vi "New Fixture.vi"() -> ()   [LabVIEW 2011]
panel:
  out "u2":bool
  out "update_1":string
  out "path_ref":refnum<vi>[](array[refnum])
  out "fixture_read":string
  out "fileexist":bool
  out "fixture":string
  out "3":bool
  out "2":bool
  out "1":bool
  in  "S4P40G":string
  in  "S4P27G":string
  in  "S4P20G":string
  out "graph_ref":refnum<vi>[](array[refnum])
  out "str_ref":refnum<vi>[](array[refnum])
  in  "S4P10G":string
  in  "Tap":enum32{"General", "Fixture Information"}(tab)
  in  "S4P Save?":bool
  in  "Rev:":string="A"
  in  "PCBPN:":string="120-000006H-048R"
  in  "Owner:":string="Shuangfeng yuan"
  in  "LifeCycle: (次)":string="3000"
  in  "Query":bool
  in  "Update":bool
  in  "Delete":bool
  in  "Save":bool
  in  "Local":bool
  in  "FixtureNo:":string="SFP+ 002"
  in  "Type:":string="SFP+"
  in  "Fixture Description:":string="SFP+ Cable Evaluation Board"
  in  "Count:":string="0"
  in  "Summary:":string
  in  "Excute":bool
  in  "40G":path
  in  "27G":path
  in  "20G":path
  in  "10G":path
  out "Delay(ns)":dbl
  in  "From File":bool
  out "Delay":T1(graph)
  out "Insertion Loss":T1(graph)
  in  "Count(invisible)":string
  in  "FixtureType":string
  in  "FixtureNo":string
  in  "FixtureRev":string
  in  "Import_FixS4P":bool caption="Start Test"
  in  "Port Type":u16(ring)
  # "SI Testing Fixture Management"
  # "Rev 1.1"
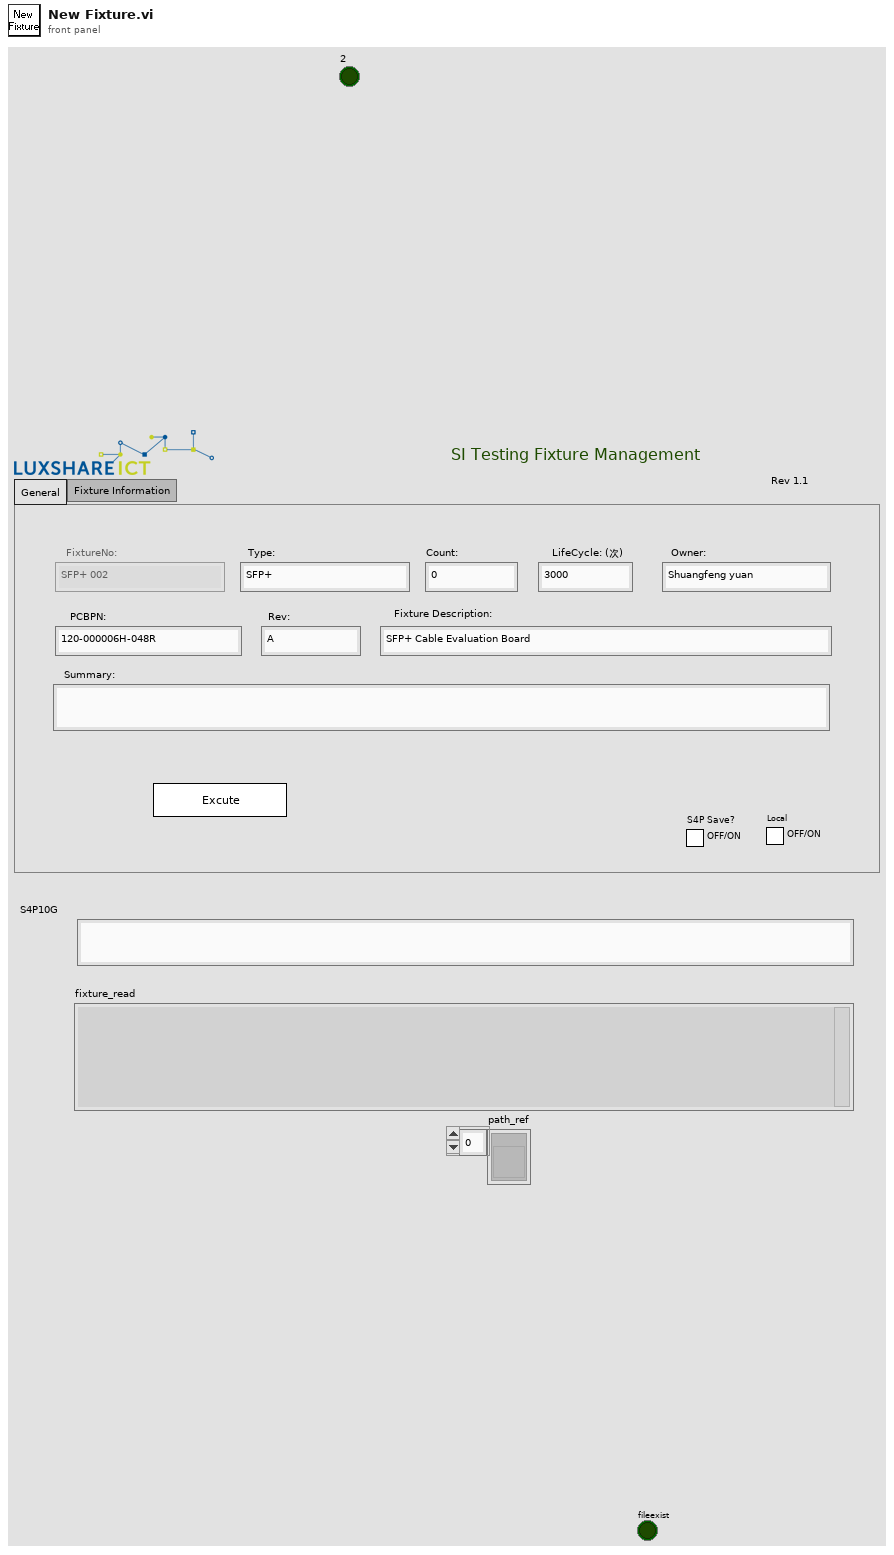
[diagram p1: front panel]
types:
  T1 = cluster{"Frequency(Hz)":dbl[], "Diff S-parameters Data":dbl[]}
  T2 = enum8{"Enabled", "Disabled", "Disabled and Grayed Out"}
  T3 = enum16{"查询表名", "查询列名", "查询记录", "查询总记录", "查询数据", "转换数据"}
  T4 = enum16{"big-endian, network order", "native, host order", "little-endian"}
  T5 = enum16{"", "创建表", "删除表", "添加表列", "删除表列", "添加数据", "删除数据"}
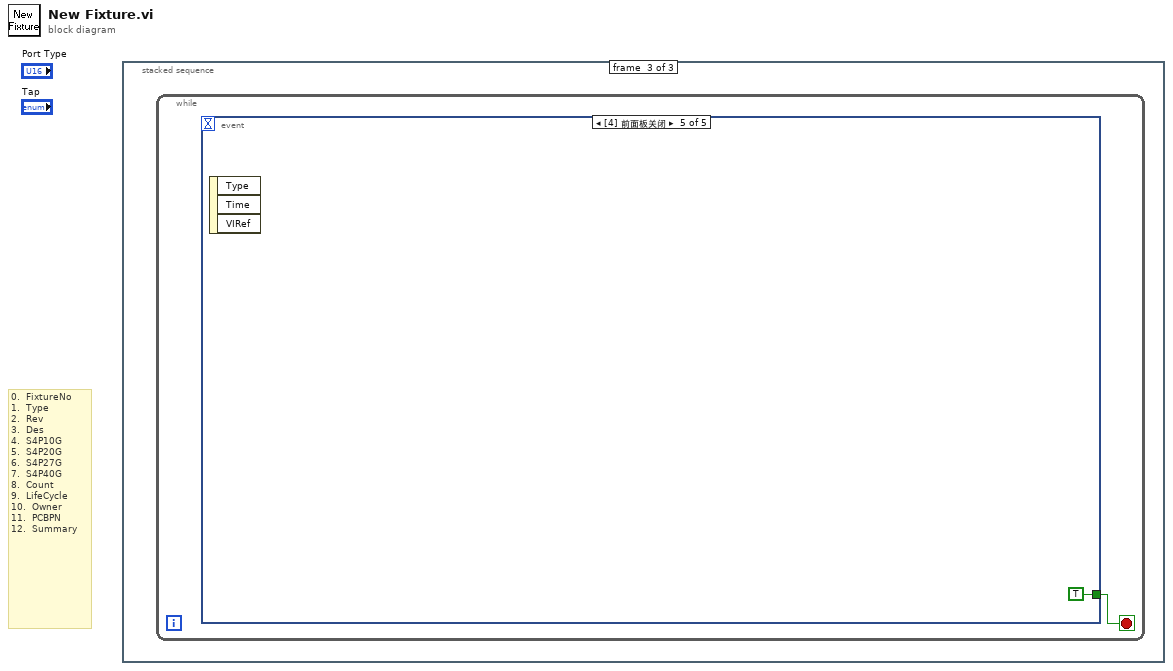
[diagram p0: block diagram]
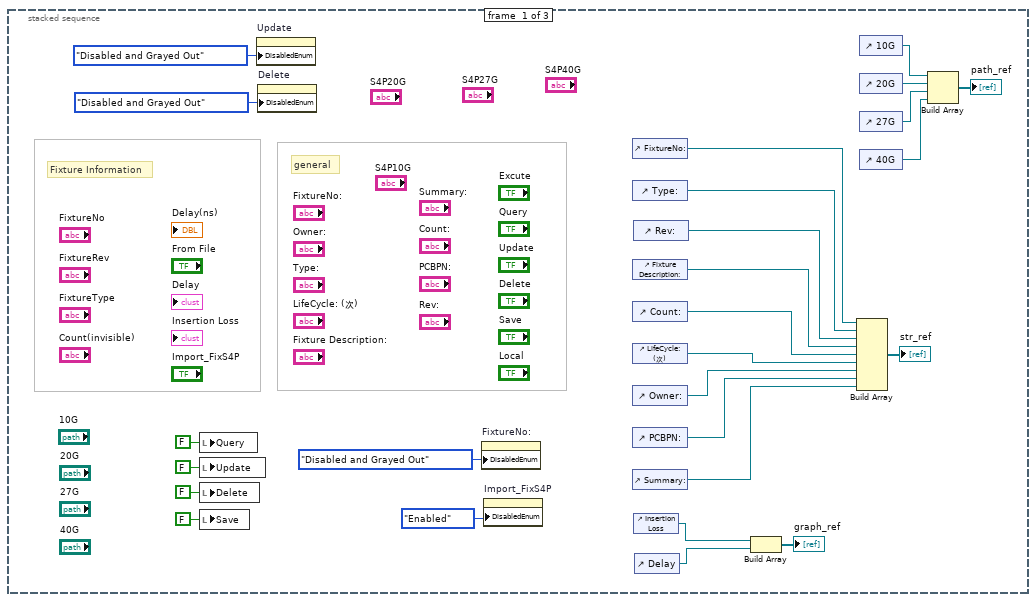
[diagram p2: hidden frame]
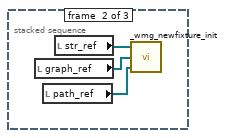
[diagram p3: hidden frame]
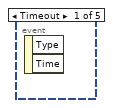
[diagram p4: hidden frame]
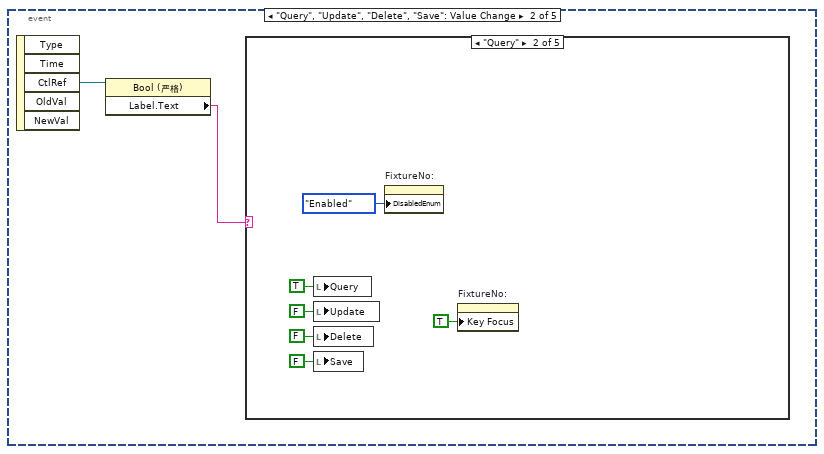
[diagram p5: hidden frame]
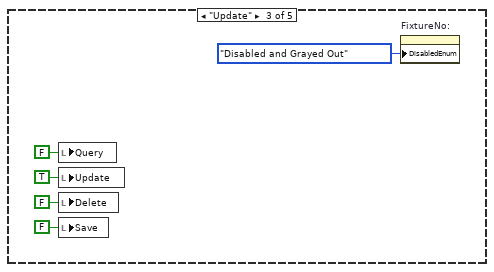
[diagram p7: hidden frame]
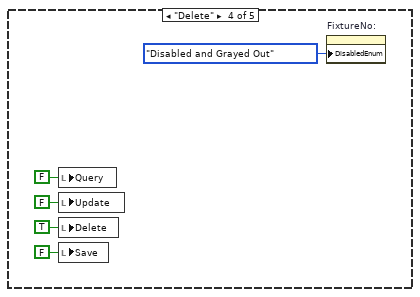
[diagram p8: hidden frame]
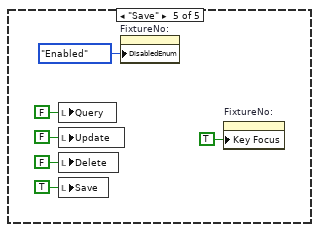
[diagram p9: hidden frame]
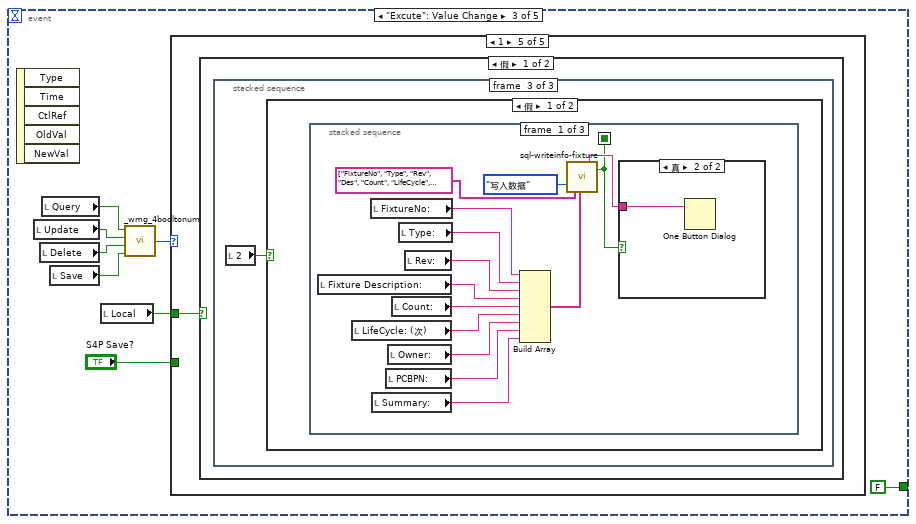
[diagram p10: hidden frame]
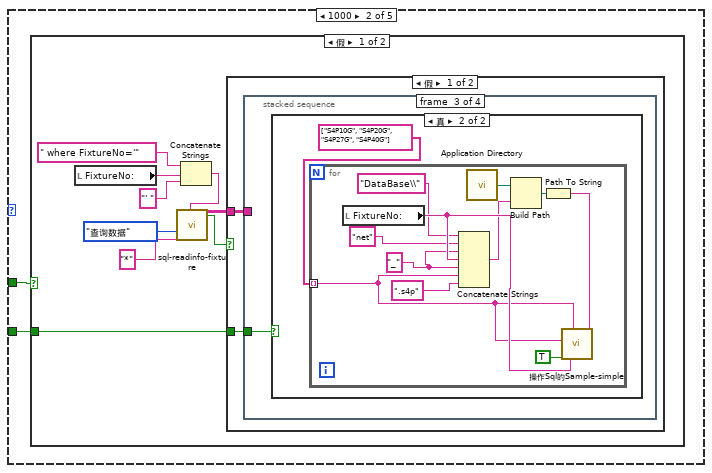
[diagram p12: hidden frame]
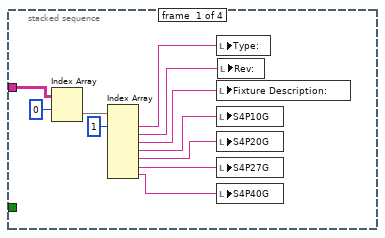
[diagram p13: hidden frame]
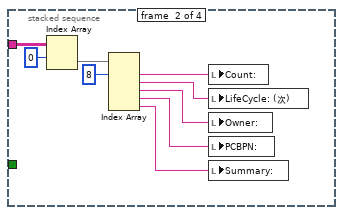
[diagram p14: hidden frame]
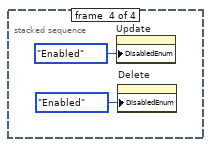
[diagram p16: hidden frame]
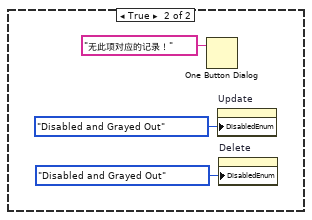
[diagram p17: hidden frame]
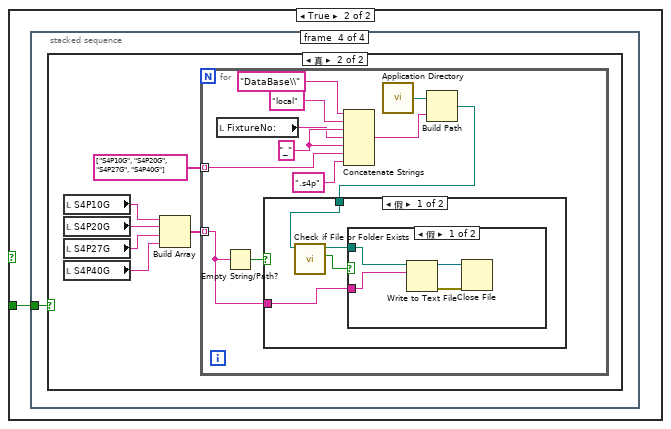
[diagram p18: hidden frame]
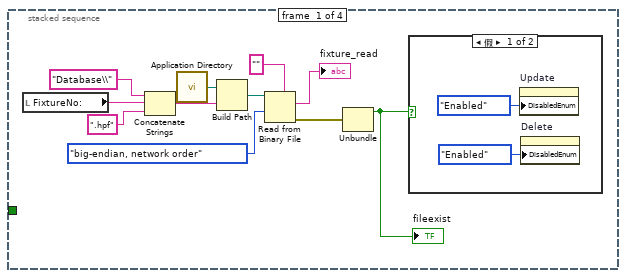
[diagram p19: hidden frame]
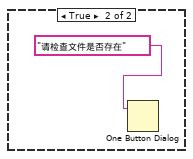
[diagram p20: hidden frame]
diagram:
  # "0.  FixtureNo\n1.  Type\n2.  Rev\n3.  Des\n4.  S4P10G\n5.  S4P20G\n6.  S4P27G\n7.  S4P40G\n8.  Count\n9.  LifeCycle\n10.  Owner\n11.  PCBPN\n12.  Summary"
  n1 = stacked-sequence {
    frame #0 {
      # "Fixture Information"
      # "general"
      n2 = local write "Query"(FALSE ("Query")) -> ()
      n3 = local write "Update"(FALSE ("Update")) -> ()
      n4 = local write "Delete"(FALSE ("Delete")) -> ()
      n5 = local write "Save"(FALSE ("Save")) -> ()
      n6 = property on="Update" class="Bool (严格)"("DisabledEnum"=T2."Disabled and Grayed Out" ("禁用")) -> ()  [unwired: 2 in, 2 out]
      n7 = property on="Delete" class="Bool (严格)"("DisabledEnum"=T2."Disabled and Grayed Out" ("禁用")) -> ()  [unwired: 2 in, 2 out]
      n8 = property on="FixtureNo:" class="Str"("DisabledEnum"=T2."Disabled and Grayed Out" ("禁用")) -> ()  [unwired: 2 in, 2 out]
      n9 = property on="Import_FixS4P" class="Bool"("DisabledEnum"=T2."Enabled" ("禁用")) -> ()  [unwired: 2 in, 2 out]
      n10 = control-ref of="FixtureNo:"() -> (w5:refnum<vi>)
      n11 = control-ref of="Type:"() -> (w4:refnum<vi>)
      n12 = control-ref of="Fixture Description:"() -> (w26:refnum<vi>)
      n13 = control-ref of="Count:"() -> (w25:refnum<vi>)
      n14 = control-ref of="LifeCycle: (次)"() -> (w24:refnum<vi>)
      n15 = control-ref of="Owner:"() -> (w23:refnum<vi>)
      n16 = control-ref of="PCBPN:"() -> (w22:refnum<vi>)
      n17 = control-ref of="Summary:"() -> (w21:refnum<vi>)
      n18 = control-ref of="Rev:"() -> (w3:refnum<vi>)
      n19 = control-ref of="Insertion Loss"() -> (w18:refnum<vi>)
      n20 = control-ref of="Delay"() -> (w17:refnum<vi>)
      n21 = Build Array(w18, w17) -> (→"graph_ref":refnum<vi>[])
      n22 = Build Array(w5, w4, w3, w26, w25, w24, w23, w22, w21) -> (→"str_ref":refnum<vi>[])
      n23 = control-ref of="10G"() -> (w10:refnum<vi>)
      n24 = control-ref of="20G"() -> (w9:refnum<vi>)
      n25 = control-ref of="27G"() -> (w8:refnum<vi>)
      n26 = control-ref of="40G"() -> (w7:refnum<vi>)
      n27 = Build Array(w10, w9, w8, w7) -> (→"path_ref":refnum<vi>[])
    }
    frame #1 {
      n28 = local read "graph_ref"() -> (w29:refnum<vi>[])
      n29 = local read "path_ref"() -> (w27:refnum<vi>[])
      n30 = local read "str_ref"() -> (w28:refnum<vi>[])
      n31 = call "_wmg_newfixture_init.vi"("path_ref"=w27, "graph_ref"=w29, "str_ref"=w28) -> ()  [unwired: 1 in]
    }
    frame #2 {
      n32 = while {
        stop <- w30 stop-if-true
        n33 = event shown="[4] 前面板关闭" {
          selector: _ -> [_ _ _ _ _]
          dyn-events: _ -> [_ _ _ _ _]
          timeout: _ -> [_ _ _ _ _]
          tunnel: [_ _ FALSE _ TRUE] -> w30
          event Timeout {
            n34 = event-data() -> ()  [unwired: 1 in, 2 out]
          }
          event "Query", "Update", "Delete", "Save": Value Change {
            n35 = event-data() -> ("CtlRef"=w32:refnum<vi>)  [unwired: 1 in, 4 out]
            n36 = property class="Bool (严格)"(reference=w32) -> ("Label.Text"=w31:string)  [unwired: 1 in, 2 out]
            n37 = case shown="\"Query\"" w31 {
              frame "假", Default {
              }
              frame "Query" {
                n38 = local write "Query"(TRUE ("Query")) -> ()
                n39 = local write "Update"(FALSE ("Update")) -> ()
                n40 = local write "Delete"(FALSE ("Delete")) -> ()
                n41 = local write "Save"(FALSE ("Save")) -> ()
                n42 = property on="FixtureNo:" class="Str"("DisabledEnum"=T2."Enabled" ("禁用")) -> ()  [unwired: 2 in, 2 out]
                n43 = property on="FixtureNo:" class="Str"("Key Focus"=TRUE ("键选中")) -> ()  [unwired: 2 in, 2 out]
              }
              frame "Update" {
                n44 = local write "Query"(FALSE ("Query")) -> ()
                n45 = local write "Update"(TRUE ("Update")) -> ()
                n46 = local write "Delete"(FALSE ("Delete")) -> ()
                n47 = local write "Save"(FALSE ("Save")) -> ()
                n48 = property on="FixtureNo:" class="Str"("DisabledEnum"=T2."Disabled and Grayed Out" ("禁用")) -> ()  [unwired: 2 in, 2 out]
              }
              frame "Delete" {
                n49 = local write "Query"(FALSE ("Query")) -> ()
                n50 = local write "Update"(FALSE ("Update")) -> ()
                n51 = local write "Delete"(TRUE ("Delete")) -> ()
                n52 = local write "Save"(FALSE ("Save")) -> ()
                n53 = property on="FixtureNo:" class="Str"("DisabledEnum"=T2."Disabled and Grayed Out" ("禁用")) -> ()  [unwired: 2 in, 2 out]
              }
              frame "Save" {
                n54 = local write "Query"(FALSE ("Query")) -> ()
                n55 = local write "Update"(FALSE ("Update")) -> ()
                n56 = local write "Delete"(FALSE ("Delete")) -> ()
                n57 = local write "Save"(TRUE ("Save")) -> ()
                n58 = property on="FixtureNo:" class="Str"("DisabledEnum"=T2."Enabled" ("禁用")) -> ()  [unwired: 2 in, 2 out]
                n59 = property on="FixtureNo:" class="Str"("Key Focus"=TRUE ("键选中")) -> ()  [unwired: 2 in, 2 out]
              }
            }
          }
          event "Excute": Value Change {
            n60 = event-data() -> ()  [unwired: 1 in, 5 out]
            n61 = local read "Update"() -> (w61:bool)
            n62 = local read "Delete"() -> (w60:bool)
            n63 = local read "Query"() -> (w62:bool)
            n64 = local read "Save"() -> (w59:bool)
            n65 = local read "Local"() -> (w57:bool)
            n66 = call "_wmg_4booltonum.vi"("input4"=w59, "input3"=w60, "input2"=w61, "input1"=w62) -> ("output"=w58:i16)
            n67 = case shown="1" w58 {
              tunnel: w57 -> [_ w64 w185 w294 w319]
              tunnel: "S4P Save?" -> [_ w63 _ _ _]
              frame 0, Default {
              }
              frame 1000 {
                n68 = case shown="假" w64 {
                  tunnel: w63 -> [w65 w114]
                  frame False {
                    n69 = local read "FixtureNo:"() -> (w73:string)
                    n70 = Concatenate Strings(" where FixtureNo='" ("限定条件"), w73, "' ") -> (w70:string)
                    n71 = call "sql-readinfo-fixture.vi"("操作模式"=T3."查询数据", "查询项目"="*", "限定条件"=w70) -> ("ConvertToArray"=w67:string[][], "status"=w66:bool)  [unwired: 14 in, 9 out]
                    n72 = case shown="假" w66 {
                      tunnel: w67 -> [w75 _]
                      tunnel: w65 -> [w74 _]
                      frame False {
                        n73 = stacked-sequence {
                          tunnel: w75 -> [w86 w94 _ _]
                          tunnel: w74 -> [_ _ w96 _]
                          frame #0 {
                            n74 = Index Array(array=w86, index (row)=0 ("索引 (行)")) -> (element=w84:string[])  [unwired: 1 in]
                            n75 = Index Array(array=w84, index #1=1 ("索引")) -> (element #1=w77:string, element #2=w76:string, element #3=w82:string, element #4=w81:string, element #5=w80:string, element #6=w79:string, element #7=w78:string)  [unwired: 6 in]
                            n76 = local write "Type:"(w77) -> ()
                            n77 = local write "Fixture Description:"(w82) -> ()
                            n78 = local write "S4P10G"(w81) -> ()
                            n79 = local write "S4P20G"(w80) -> ()
                            n80 = local write "S4P27G"(w79) -> ()
                            n81 = local write "S4P40G"(w78) -> ()
                            n82 = local write "Rev:"(w76) -> ()
                          }
                          frame #1 {
                            n83 = Index Array(array=w94, index (row)=0 ("索引 (行)")) -> (element=w93:string[])  [unwired: 1 in]
                            n84 = Index Array(array=w93, index #1=8 ("索引")) -> (element #1=w91:string, element #2=w90:string, element #3=w89:string, element #4=w88:string, element #5=w87:string)  [unwired: 4 in]
                            n85 = local write "Count:"(w91) -> ()
                            n86 = local write "LifeCycle: (次)"(w90) -> ()
                            n87 = local write "Owner:"(w89) -> ()
                            n88 = local write "PCBPN:"(w88) -> ()
                            n89 = local write "Summary:"(w87) -> ()
                          }
                          frame #2 {
                            n90 = case shown="真" w96 {
                              frame False {
                              }
                              frame True {
                                n91 = for {
                                tunnel: string[] ["S4P10G", "S4P20G", "S4P27G", "S4P40G"] -> [w107] mode=indexing
                                w98 = "_"
                                n92 = local read "FixtureNo:"() -> (w108:string)
                                n93 = Concatenate Strings("DataBase\\" ("字符串"), "net", w98, w108, w98, w107, ".s4p" ("字符串")) -> (w103:string)
                                n94 = call <vilib>:"Application Directory.vi"() -> ("Application Directory"=w106:path)
                                n95 = Build Path(base path=w106, name or relative path=w103) -> (appended path=w102:path)
                                n96 = Path To String(path=w102) -> (string=w101:string)
                                n97 = call "操作Sql的Sample-simple.vi"("SavefileName"=w101, "sn 2"=w108, "fieldName"=w107, "下载文件"=TRUE, "fieldName_Index"=w107) -> ()  [unwired: 7 in]
                                }
                              }
                            }
                          }
                          frame #3 {
                            n98 = property on="Update" class="Bool (严格)"("DisabledEnum"=T2."Enabled" ("禁用")) -> ()  [unwired: 2 in, 2 out]
                            n99 = property on="Delete" class="Bool (严格)"("DisabledEnum"=T2."Enabled" ("禁用")) -> ()  [unwired: 2 in, 2 out]
                          }
                        }
                      }
                      frame True {
                        n100 = One Button Dialog(message="无此项对应的记录！" ("消息")) -> ()  [unwired: 1 in, 1 out]
                        n101 = property on="Update" class="Bool (严格)"("DisabledEnum"=T2."Disabled and Grayed Out" ("禁用")) -> ()  [unwired: 2 in, 2 out]
                        n102 = property on="Delete" class="Bool (严格)"("DisabledEnum"=T2."Disabled and Grayed Out" ("禁用")) -> ()  [unwired: 2 in, 2 out]
                      }
                    }
                  }
                  frame True {
                    n103 = stacked-sequence {
                      tunnel: w114 -> [_ _ _ w154]
                      frame #0 {
                        n104 = local read "FixtureNo:"() -> (w117:string)
                        n105 = Concatenate Strings("Database\\" ("字符串"), w117, ".hpf") -> (w120:string)
                        n106 = call <vilib>:"Application Directory.vi"() -> ("Application Directory"=w119:path)
                        n107 = Build Path(base path=w119, name or relative path=w120) -> (appended path=w121:path)
                        n108 = Read from Binary File(5:"" ("数据类型"), 9:T4."big-endian, network order" ("字节顺序(0:big-endian, network order)"), 11:w121) -> (0:w124:errorcluster, 2:→"fixture_read":string)  [unwired: 3 in, 2 out]
                        n109 = Unbundle(w124) -> ("status"=w125:bool)  [unwired: 2 out]
                        "fileexist" <- w125
                        n110 = case shown="假" w125 {
                          frame False {
                            n111 = property on="Update" class="Bool (严格)"("DisabledEnum"=T2."Enabled" ("禁用")) -> ()  [unwired: 2 in, 2 out]
                            n112 = property on="Delete" class="Bool (严格)"("DisabledEnum"=T2."Enabled" ("禁用")) -> ()  [unwired: 2 in, 2 out]
                          }
                          frame True {
                            n113 = One Button Dialog(message="请检查文件是否存在") -> ()  [unwired: 1 in, 1 out]
                          }
                        }
                      }
                      frame #1 {
                        n114 = local read "fixture_read"() -> (w142:string)
                        n115 = Spreadsheet String To Array(delimiter (Tab)="@" ("分隔符(Tab)"), format string="" ("格式字符串"), spreadsheet string=w142, array type (2D Dbl)=string[] []) -> (array=w141:string[])
                        n116 = Index Array(array=w141, index #1=1 ("索引"), index #4=8 ("索引")) -> (element #1=w131:string, element #2=w129:string, element #3=w130:string, element #4=w138:string, element #5=w137:string, element #6=w136:string, element #7=w135:string, element #8=w134:string)  [unwired: 6 in]
                        n117 = local write "Type:"(w131) -> ()
                        n118 = local write "Fixture Description:"(w130) -> ()
                        n119 = local write "Count:"(w138) -> ()
                        n120 = local write "LifeCycle: (次)"(w137) -> ()
                        n121 = local write "Owner:"(w136) -> ()
                        n122 = local write "PCBPN:"(w135) -> ()
                        n123 = local write "Summary:"(w134) -> ()
                        n124 = local write "Rev:"(w129) -> ()
                      }
                      frame #2 {
                        n125 = local read "fixture_read"() -> (w152:string)
                        n126 = Spreadsheet String To Array(delimiter (Tab)="@" ("分隔符(Tab)"), format string="" ("格式字符串"), spreadsheet string=w152, array type (2D Dbl)=string[] []) -> (array=w151:string[])
                        n127 = Index Array(array=w151, index #1=4 ("索引")) -> (element #1=w147:string, element #2=w146:string, element #3=w145:string, element #4=w144:string)  [unwired: 3 in]
                        n128 = local write "S4P10G"(w147) -> ()
                        n129 = local write "S4P20G"(w146) -> ()
                        n130 = local write "S4P27G"(w145) -> ()
                        n131 = local write "S4P40G"(w144) -> ()
                      }
                      frame #3 {
                        n132 = case shown="真" w154 {
                          frame False {
                          }
                          frame True {
                            n133 = local read "S4P10G"() -> (w160:string)
                            n134 = local read "S4P20G"() -> (w159:string)
                            n135 = local read "S4P27G"() -> (w158:string)
                            n136 = local read "S4P40G"() -> (w157:string)
                            n137 = Build Array(w160, w159, w158, w157) -> (w156:string[])
                            n138 = for {
                              tunnel: w156 -> [w166] mode=indexing
                              tunnel: string[] ["S4P10G", "S4P20G", "S4P27G", "S4P40G"] -> [w161] mode=indexing
                              w163 = "_"
                              n139 = local read "FixtureNo:"() -> (w162:string)
                              n140 = Empty String/Path?(string/path=w166) -> (empty?=w171:bool)
                              n141 = Concatenate Strings("DataBase\\" ("字符串"), "local" ("字符串"), w163, w162, w163, w161, ".s4p" ("字符串")) -> (w168:string)
                              n142 = call <vilib>:"Application Directory.vi"() -> ("Application Directory"=w170:path)
                              n143 = Build Path(base path=w170, name or relative path=w168) -> (appended path=w167:path)
                              n144 = case shown="假" w171 {
                                tunnel: w167 -> [w175 _]
                                tunnel: w166 -> [w172 _]
                                frame False {
                                n145 = call <vilib>:"Check if File or Folder Exists.vi"("path"=w175) -> ("file or folder exists?"=w174:bool, "dup path"=w173:path)  [unwired: 8 in, 1 out]
                                n146 = case shown="假" w174 {
                                tunnel: w173 -> [w179 w182]
                                tunnel: w172 -> [w178 w183]
                                frame False {
                                n147 = Write to Text File(file (use dialog)=w179, text=w178) -> (refnum out=w176:refnum<file>, error out=w177:errorcluster)  [unwired: 2 in, 1 out]
                                n148 = Close File(refnum=w176, error in=w177) -> ()  [unwired: 2 out]
                                }
                                frame True {
                                n149 = Delete(path (use dialog)=w182) -> (deleted path=w184:path)  [unwired: 4 in, 2 out]
                                n150 = Write to Text File(file (use dialog)=w184, text=w183) -> (refnum out=w180:refnum<file>, error out=w181:errorcluster)  [unwired: 2 in, 1 out]
                                n151 = Close File(refnum=w180, error in=w181) -> ()  [unwired: 2 out]
                                }
                                }
                                }
                                frame True {
                                }
                              }
                            }
                          }
                        }
                      }
                    }
                  }
                }
              }
              frame 100 {
                n152 = case shown="假" w185 {
                  frame False {
                    n153 = stacked-sequence {
                      frame #0 {
                        n154 = stacked-sequence {
                          frame #0 {
                            n155 = local read "10G"() -> (w187:path)
                            n156 = call "_wmg_readFile.vi"("路径"=w187) -> ("字符串"=w186:string)
                            n157 = local write "S4P10G"(w186) -> ()
                          }
                          frame #1 {
                            n158 = local read "20G"() -> (w189:path)
                            n159 = call "_wmg_readFile.vi"("路径"=w189) -> ("字符串"=w188:string)
                            n160 = local write "S4P20G"(w188) -> ()
                          }
                          frame #2 {
                            n161 = local read "27G"() -> (w191:path)
                            n162 = call "_wmg_readFile.vi"("路径"=w191) -> ("字符串"=w190:string)
                            n163 = local write "S4P27G"(w190) -> ()
                          }
                          frame #3 {
                            n164 = local read "40G"() -> (w193:path)
                            n165 = call "_wmg_readFile.vi"("路径"=w193) -> ("字符串"=w192:string)
                            n166 = local write "S4P40G"(w192) -> ()
                          }
                        }
                      }
                      frame #1 {
                        n167 = local read "S4P10G"() -> (w202:string)
                        n168 = local read "S4P20G"() -> (w201:string)
                        n169 = local read "S4P27G"() -> (w200:string)
                        n170 = local read "S4P40G"() -> (w199:string)
                        n171 = Empty String/Path?(string/path=w200) -> (empty?=w196:bool)
                        n172 = Empty String/Path?(string/path=w199) -> (empty?=w195:bool)
                        n173 = Empty String/Path?(string/path=w202) -> (empty?=w198:bool)
                        n174 = Empty String/Path?(string/path=w201) -> (empty?=w197:bool)
                        n175 = Compound Arithmetic op=AND(w198, w197, w196, w195) -> (→"1":bool)
                      }
                      frame #2 {
                        n176 = local read "1"() -> (w203:bool)
                        n177 = case shown="假" w203 {
                          frame False {
                            n178 = stacked-sequence {
                              seq-local: [w204 _ _] -> [_ _ w239]
                              frame #0 {
                                n179 = local read "Fixture Description:"() -> (w209:string)
                                n180 = local read "LifeCycle: (次)"() -> (w220:string)
                                n181 = local read "Summary:"() -> (w217:string)
                                n182 = local read "FixtureNo:"() -> (w214:string)
                                n183 = local read "PCBPN:"() -> (w218:string)
                                n184 = local read "Owner:"() -> (w219:string)
                                n185 = local read "Count:"() -> (w221:string)
                                n186 = local read "Type:"() -> (w210:string)
                                n187 = local read "Rev:"() -> (w208:string)
                                n188 = Concatenate Strings(" where FixtureNo='" ("限定条件"), w214, "' ") -> (w211:string)
                                n189 = Build Array(w210, w208, w209, w221, w220, w219, w218, w217) -> (w206:string[])
                                n190 = call "_wmg_updateItemConValue.vi"("Values"=w206, "Items"=string[] ["Type", "Rev", "Des", "Count", "LifeCycle", "Owner", "PCBPN", "Summary"]) -> ("Output"=w205:string)
                                n191 = call "sql-writeinfo-fixture.vi"("操作模式"=enum16{"写入数据", "更改数据"}."更改数据", "设置"=w205, "条件"=w211) -> ("简单报错"=w216:string, "status"=w204:bool)  [unwired: 15 in]
                                n192 = case shown="真" w204 {
                                tunnel: w216 -> [_ w223]
                                frame False {
                                n193 = One Button Dialog(message="数据更新成功！") -> ()  [unwired: 1 in, 1 out]
                                }
                                frame True {
                                n194 = One Button Dialog(message=w223) -> ()  [unwired: 1 in, 1 out]
                                }
                                }
                              }
                              frame #1 {
                                n195 = local read "10G"() -> (w226:path)
                                n196 = local read "20G"() -> (w227:path)
                                n197 = local read "27G"() -> (w228:path)
                                n198 = local read "40G"() -> (w229:path)
                                n199 = Build Array(w226, w227, w228, w229) -> (w225:path[])
                                n200 = for {
                                tunnel: w225 -> [w234] mode=indexing
                                tunnel: string[] ["S4P10G", "S4P20G", "S4P27G", "S4P40G"] -> [w231] mode=indexing
                                n201 = local read "FixtureNo:"() -> (w232:string)
                                n202 = Path To String(path=w234) -> (string=w233:string)
                                n203 = Empty String/Path?(string/path=w234) -> (empty?=w230:bool)
                                n204 = case shown="假" w230 {
                                tunnel: w233 -> [w237 _]
                                tunnel: w232 -> [w236 _]
                                tunnel: w231 -> [w235 _]
                                frame False {
                                n205 = call "操作Sql的Sample-simple.vi"("下载文件"=FALSE, "fileName"=w237, "fieldName_Index"=w235, "sn"=w236) -> ()  [unwired: 8 in]
                                }
                                frame True {
                                }
                                }
                                }
                              }
                              frame #2 {
                                n206 = case shown="假" w239 {
                                frame False {
                                n207 = local read "graph_ref"() -> (w242:refnum<vi>[])
                                n208 = local read "path_ref"() -> (w240:refnum<vi>[])
                                n209 = local read "str_ref"() -> (w241:refnum<vi>[])
                                n210 = call "_wmg_newfixture_init.vi"("path_ref"=w240, "graph_ref"=w242, "str_ref"=w241) -> ()  [unwired: 1 in]
                                }
                                frame True {
                                }
                                }
                              }
                            }
                          }
                          frame True {
                            n211 = One Button Dialog(message="S4P至少要一个不为空！" ("消息")) -> ()  [unwired: 1 in, 1 out]
                          }
                        }
                      }
                    }
                  }
                  frame True {
                    n212 = stacked-sequence {
                      frame #0 {
                        n213 = stacked-sequence {
                          frame #0 {
                            n214 = local read "10G"() -> (w245:path)
                            n215 = call "_wmg_readFile.vi"("路径"=w245) -> ("字符串"=w244:string)
                            n216 = local write "S4P10G"(w244) -> ()
                          }
                          frame #1 {
                            n217 = local read "20G"() -> (w247:path)
                            n218 = call "_wmg_readFile.vi"("路径"=w247) -> ("字符串"=w246:string)
                            n219 = local write "S4P20G"(w246) -> ()
                          }
                          frame #2 {
                            n220 = local read "27G"() -> (w249:path)
                            n221 = call "_wmg_readFile.vi"("路径"=w249) -> ("字符串"=w248:string)
                            n222 = local write "S4P27G"(w248) -> ()
                          }
                          frame #3 {
                            n223 = local read "40G"() -> (w251:path)
                            n224 = call "_wmg_readFile.vi"("路径"=w251) -> ("字符串"=w250:string)
                            n225 = local write "S4P40G"(w250) -> ()
                          }
                        }
                      }
                      frame #1 {
                        n226 = local read "S4P10G"() -> (w259:string)
                        n227 = local read "S4P20G"() -> (w258:string)
                        n228 = local read "S4P27G"() -> (w257:string)
                        n229 = local read "S4P40G"() -> (w256:string)
                        n230 = Empty String/Path?(string/path=w257) -> (empty?=w253:bool)
                        n231 = Empty String/Path?(string/path=w256) -> (empty?=w252:bool)
                        n232 = Empty String/Path?(string/path=w259) -> (empty?=w255:bool)
                        n233 = Empty String/Path?(string/path=w258) -> (empty?=w254:bool)
                        n234 = Compound Arithmetic op=AND(w255, w254, w253, w252) -> (→"u2":bool)
                      }
                      frame #2 {
                        n235 = local read "S4P10G"() -> (w276:string)
                        n236 = local read "S4P20G"() -> (w275:string)
                        n237 = local read "S4P27G"() -> (w274:string)
                        n238 = local read "S4P40G"() -> (w273:string)
                        n239 = local read "Fixture Description:"() -> (w277:string)
                        n240 = local read "LifeCycle: (次)"() -> (w271:string)
                        n241 = local read "Summary:"() -> (w268:string)
                        n242 = local read "PCBPN:"() -> (w269:string)
                        n243 = local read "Owner:"() -> (w270:string)
                        n244 = local read "Count:"() -> (w272:string)
                        n245 = local read "FixtureNo:"() -> (w264:string)
                        n246 = local read "Type:"() -> (w263:string)
                        n247 = local read "Rev:"() -> (w262:string)
                        n248 = Build Array(w264, w263, w262, w277, w276, w275, w274, w273, w272, w271, w270, w269, w268) -> (w267:string[])
                        n249 = Array To Spreadsheet String(delimiter (Tab)="@" ("分隔符(Tab)"), array=w267, 3:"" ("格式字符串")) -> (spreadsheet string=→"update_1":string)
                      }
                      frame #3 {
                        n250 = local read "u2"() -> (w278:bool)
                        n251 = case shown="假" w278 {
                          frame False {
                            n252 = stacked-sequence {
                              frame #0 {
                                n253 = local read "FixtureNo:"() -> (w282:string)
                                n254 = local read "update_1"() -> (w281:string)
                                n255 = call <vilib>:"Application Directory.vi"() -> ("Application Directory"=w283:path)
                                n256 = Concatenate Strings("Database\\" ("字符串"), w282, ".hpf" ("字符串")) -> (w284:string)
                                n257 = Build Path(base path=w283, name or relative path=w284) -> (appended path=w288:path)
                                n258 = Write to Binary File(file (use dialog)=w288, data=w281, 9:T4."big-endian, network order" ("字节顺序(0:big-endian, network order)")) -> (refnum out=w279:refnum<file>, error out=w280:errorcluster)  [unwired: 3 in, 1 out]
                                n259 = Close File(refnum=w279, error in=w280) -> ()  [unwired: 2 out]
                              }
                              frame #1 {
                                n260 = local read "graph_ref"() -> (w292:refnum<vi>[])
                                n261 = local read "path_ref"() -> (w290:refnum<vi>[])
                                n262 = local read "str_ref"() -> (w291:refnum<vi>[])
                                n263 = call "_wmg_newfixture_init.vi"("path_ref"=w290, "graph_ref"=w292, "str_ref"=w291) -> ()  [unwired: 1 in]
                                n264 = One Button Dialog(message="文件更新成功！") -> ()  [unwired: 1 in, 1 out]
                              }
                            }
                          }
                          frame True {
                            n265 = One Button Dialog(message="S4P至少要一个不为空！" ("消息")) -> ()  [unwired: 1 in, 1 out]
                          }
                        }
                      }
                    }
                  }
                }
              }
              frame 10 {
                n266 = case shown="假" w294 {
                  frame False {
                    n267 = stacked-sequence {
                      frame #0 {
                        n268 = local read "FixtureNo:"() -> (w300:string)
                        n269 = Concatenate Strings(" where FixtureNo='" ("限定条件"), w300, "' ") -> (w297:string)
                        n270 = call "sql-delete-fixture.vi"("操作模式"=T5."删除数据", "限定条件"=w297) -> ("错误类型"=w295:string, "status"=w296:bool)  [unwired: 16 in]
                        n271 = case shown="假" w296 {
                          tunnel: w295 -> [_ w303]
                          frame False {
                            n272 = One Button Dialog(message="数据删除成功！") -> ()  [unwired: 1 in, 1 out]
                          }
                          frame True {
                            n273 = One Button Dialog(message=w303) -> ()  [unwired: 1 in, 1 out]
                          }
                        }
                      }
                      frame #1 {
                        n274 = local read "graph_ref"() -> (w306:refnum<vi>[])
                        n275 = local read "path_ref"() -> (w304:refnum<vi>[])
                        n276 = local read "str_ref"() -> (w305:refnum<vi>[])
                        n277 = call "_wmg_newfixture_init.vi"("path_ref"=w304, "graph_ref"=w306, "str_ref"=w305) -> ()  [unwired: 1 in]
                      }
                    }
                  }
                  frame True {
                    n278 = local read "FixtureNo:"() -> (w311:string)
                    n279 = call <vilib>:"Application Directory.vi"() -> ("Application Directory"=w307:path)
                    n280 = Concatenate Strings("Database\\" ("字符串"), w311, ".hpj" ("字符串")) -> (w308:string)
                    n281 = Build Path(base path=w307, name or relative path=w308) -> (appended path=w312:path)
                    n282 = Delete(path (use dialog)=w312) -> (error out=w316:errorcluster)  [unwired: 4 in, 2 out]
                    n283 = Unbundle(w316) -> ("status"=w313:bool, "source"=w315:string)  [unwired: 1 out]
                    n284 = case shown="假" w313 {
                      tunnel: ["文件删除成功！" ("消息") w318] -> w314
                      tunnel: w315 -> [_ w318]
                      frame False {
                      }
                      frame True {
                      }
                    }
                    n285 = One Button Dialog(message=w314) -> ()  [unwired: 1 in, 1 out]
                  }
                }
              }
              frame 1 {
                n286 = case shown="假" w319 {
                  frame False {
                    n287 = stacked-sequence {
                      frame #0 {
                        n288 = stacked-sequence {
                          frame #0 {
                            n289 = local read "10G"() -> (w321:path)
                            n290 = call "_wmg_readFile.vi"("路径"=w321) -> ("字符串"=w320:string)
                            n291 = local write "S4P10G"(w320) -> ()
                          }
                          frame #1 {
                            n292 = local read "20G"() -> (w323:path)
                            n293 = call "_wmg_readFile.vi"("路径"=w323) -> ("字符串"=w322:string)
                            n294 = local write "S4P20G"(w322) -> ()
                          }
                          frame #2 {
                            n295 = local read "27G"() -> (w325:path)
                            n296 = call "_wmg_readFile.vi"("路径"=w325) -> ("字符串"=w324:string)
                            n297 = local write "S4P27G"(w324) -> ()
                          }
                          frame #3 {
                            n298 = local read "40G"() -> (w327:path)
                            n299 = call "_wmg_readFile.vi"("路径"=w327) -> ("字符串"=w326:string)
                            n300 = local write "S4P40G"(w326) -> ()
                          }
                        }
                      }
                      frame #1 {
                        n301 = local read "S4P10G"() -> (w336:string)
                        n302 = local read "S4P20G"() -> (w335:string)
                        n303 = local read "S4P27G"() -> (w334:string)
                        n304 = local read "S4P40G"() -> (w333:string)
                        n305 = Empty String/Path?(string/path=w334) -> (empty?=w330:bool)
                        n306 = Empty String/Path?(string/path=w333) -> (empty?=w329:bool)
                        n307 = Empty String/Path?(string/path=w336) -> (empty?=w332:bool)
                        n308 = Empty String/Path?(string/path=w335) -> (empty?=w331:bool)
                        n309 = Compound Arithmetic op=AND(w332, w331, w330, w329) -> (→"2":bool)
                      }
                      frame #2 {
                        n310 = local read "2"() -> (w337:bool)
                        n311 = case shown="假" w337 {
                          frame False {
                            n312 = stacked-sequence {
                              seq-local: [w338 _ _] -> [_ _ w369]
                              frame #0 {
                                n313 = local read "Fixture Description:"() -> (w341:string)
                                n314 = local read "LifeCycle: (次)"() -> (w350:string)
                                n315 = local read "FixtureNo:"() -> (w343:string)
                                n316 = local read "Summary:"() -> (w347:string)
                                n317 = local read "PCBPN:"() -> (w348:string)
                                n318 = local read "Owner:"() -> (w349:string)
                                n319 = local read "Count:"() -> (w351:string)
                                n320 = local read "Type:"() -> (w342:string)
                                n321 = local read "Rev:"() -> (w340:string)
                                n322 = Build Array(w343, w342, w340, w341, w351, w350, w349, w348, w347) -> (w346:string[])
                                n323 = call "sql-writeinfo-fixture.vi"("操作模式"=enum16{"写入数据", "更改数据"}."写入数据", "列名"=string[] ["FixtureNo", "Type", "Rev", "Des", "Count", "LifeCycle", "Owner", "PCBPN", "Summary"], "值"=w346) -> ("简单报错"=w345:string, "status"=w338:bool)  [unwired: 15 in]
                                n324 = case shown="真" w338 {
                                tunnel: w345 -> [_ w353]
                                frame False {
                                n325 = One Button Dialog(message="操作成功！") -> ()  [unwired: 1 in, 1 out]
                                }
                                frame True {
                                n326 = One Button Dialog(message=w353) -> ()  [unwired: 1 in, 1 out]
                                }
                                }
                              }
                              frame #1 {
                                n327 = local read "10G"() -> (w356:path)
                                n328 = local read "20G"() -> (w357:path)
                                n329 = local read "27G"() -> (w358:path)
                                n330 = local read "40G"() -> (w359:path)
                                n331 = Build Array(w356, w357, w358, w359) -> (w355:path[])
                                n332 = for {
                                tunnel: w355 -> [w364] mode=indexing
                                tunnel: string[] ["S4P10G", "S4P20G", "S4P27G", "S4P40G"] -> [w361] mode=indexing
                                n333 = local read "FixtureNo:"() -> (w362:string)
                                n334 = Path To String(path=w364) -> (string=w363:string)
                                n335 = Empty String/Path?(string/path=w364) -> (empty?=w360:bool)
                                n336 = case shown="假" w360 {
                                tunnel: w363 -> [w367 _]
                                tunnel: w362 -> [w366 _]
                                tunnel: w361 -> [w365 _]
                                frame False {
                                n337 = call "操作Sql的Sample-simple.vi"("下载文件"=FALSE, "fileName"=w367, "fieldName_Index"=w365, "sn"=w366) -> ()  [unwired: 8 in]
                                }
                                frame True {
                                }
                                }
                                }
                              }
                              frame #2 {
                                n338 = case shown="假" w369 {
                                frame False {
                                n339 = local read "graph_ref"() -> (w372:refnum<vi>[])
                                n340 = local read "path_ref"() -> (w370:refnum<vi>[])
                                n341 = local read "str_ref"() -> (w371:refnum<vi>[])
                                n342 = call "_wmg_newfixture_init.vi"("path_ref"=w370, "graph_ref"=w372, "str_ref"=w371) -> ()  [unwired: 1 in]
                                }
                                frame True {
                                }
                                }
                              }
                            }
                          }
                          frame True {
                            n343 = One Button Dialog(message="Fixture的S4P文件至少要有一个！" ("消息")) -> ()  [unwired: 1 in, 1 out]
                          }
                        }
                      }
                    }
                  }
                  frame True {
                    n344 = stacked-sequence {
                      frame #0 {
                        n345 = stacked-sequence {
                          frame #0 {
                            n346 = local read "10G"() -> (w375:path)
                            n347 = call "_wmg_readFile.vi"("路径"=w375) -> ("字符串"=w374:string)
                            n348 = local write "S4P10G"(w374) -> ()
                          }
                          frame #1 {
                            n349 = local read "20G"() -> (w377:path)
                            n350 = call "_wmg_readFile.vi"("路径"=w377) -> ("字符串"=w376:string)
                            n351 = local write "S4P20G"(w376) -> ()
                          }
                          frame #2 {
                            n352 = local read "27G"() -> (w379:path)
                            n353 = call "_wmg_readFile.vi"("路径"=w379) -> ("字符串"=w378:string)
                            n354 = local write "S4P27G"(w378) -> ()
                          }
                          frame #3 {
                            n355 = local read "40G"() -> (w381:path)
                            n356 = call "_wmg_readFile.vi"("路径"=w381) -> ("字符串"=w380:string)
                            n357 = local write "S4P40G"(w380) -> ()
                          }
                        }
                      }
                      frame #1 {
                        n358 = local read "S4P10G"() -> (w390:string)
                        n359 = local read "S4P20G"() -> (w389:string)
                        n360 = local read "S4P27G"() -> (w388:string)
                        n361 = local read "S4P40G"() -> (w387:string)
                        n362 = Empty String/Path?(string/path=w388) -> (empty?=w384:bool)
                        n363 = Empty String/Path?(string/path=w387) -> (empty?=w383:bool)
                        n364 = Empty String/Path?(string/path=w390) -> (empty?=w386:bool)
                        n365 = Empty String/Path?(string/path=w389) -> (empty?=w385:bool)
                        n366 = Compound Arithmetic op=AND(w386, w385, w384, w383) -> (→"3":bool)
                      }
                      frame #2 {
                        n367 = local read "3"() -> (w391:bool)
                        n368 = case shown="假" w391 {
                          frame False {
                            n369 = stacked-sequence {
                              frame #0 {
                                n370 = local read "S4P10G"() -> (w407:string)
                                n371 = local read "S4P20G"() -> (w406:string)
                                n372 = local read "S4P27G"() -> (w405:string)
                                n373 = local read "S4P10G"() -> (w404:string)
                                n374 = local read "Fixture Description:"() -> (w408:string)
                                n375 = local read "LifeCycle: (次)"() -> (w402:string)
                                n376 = local read "Summary:"() -> (w399:string)
                                n377 = local read "PCBPN:"() -> (w400:string)
                                n378 = local read "Owner:"() -> (w401:string)
                                n379 = local read "Count:"() -> (w403:string)
                                n380 = local read "FixtureNo:"() -> (w394:string)
                                n381 = local read "Type:"() -> (w393:string)
                                n382 = local read "Rev:"() -> (w392:string)
                                n383 = Build Array(w394, w393, w392, w408, w407, w406, w405, w404, w403, w402, w401, w400, w399) -> (w398:string[])
                                n384 = Array To Spreadsheet String(delimiter (Tab)="@" ("分隔符(Tab)"), array=w398, 3:"" ("格式字符串")) -> (spreadsheet string=→"fixture":string)
                              }
                              frame #1 {
                                n385 = local read "FixtureNo:"() -> (w409:string)
                                n386 = call <vilib>:"Application Directory.vi"() -> ("Application Directory"=w412:path)
                                n387 = Concatenate Strings("Database\\" ("字符串"), w409, ".hpf" ("字符串")) -> (w413:string)
                                n388 = Build Path(base path=w412, name or relative path=w413) -> (appended path=w416:path)
                                n389 = call <vilib>:"Check if File or Folder Exists.vi"("path"=w416) -> ("file or folder exists?"=w411:bool, "dup path"=w410:path)  [unwired: 8 in, 1 out]
                                n390 = case shown="假" w411 {
                                tunnel: w410 -> [w417 w425]
                                frame False {
                                n391 = stacked-sequence {
                                tunnel: w417 -> [w418 _]
                                frame #0 {
                                n392 = local read "fixture"() -> (w419:string)
                                n393 = One Button Dialog(message="Saved successfully!" ("消息")) -> ()  [unwired: 1 in, 1 out]
                                n394 = Write to Binary File(file (use dialog)=w418, data=w419, 9:T4."big-endian, network order" ("字节顺序(0:big-endian, network order)")) -> ()  [unwired: 3 in, 3 out]
                                }
                                frame #1 {
                                n395 = local read "graph_ref"() -> (w424:refnum<vi>[])
                                n396 = local read "path_ref"() -> (w422:refnum<vi>[])
                                n397 = local read "str_ref"() -> (w423:refnum<vi>[])
                                n398 = call "_wmg_newfixture_init.vi"("path_ref"=w422, "graph_ref"=w424, "str_ref"=w423) -> ()  [unwired: 1 in]
                                }
                                }
                                }
                                frame True {
                                n399 = Two Button Dialog(message="该PN的文件已经存在\n是否覆盖？", 1:"取消" ("F按钮名称（“取消”）"), 2:"覆盖" ("T按钮名称（“确定”）")) -> (T button?=w426:bool)
                                n400 = case shown="真" w426 {
                                tunnel: w425 -> [_ w430]
                                frame False {
                                }
                                frame True {
                                n401 = stacked-sequence {
                                tunnel: w430 -> [w432 _]
                                frame #0 {
                                n402 = local read "fixture"() -> (w431:string)
                                n403 = One Button Dialog(message="Coved successfully!" ("消息")) -> ()  [unwired: 1 in, 1 out]
                                n404 = Write to Binary File(file (use dialog)=w432, data=w431, 9:T4."big-endian, network order" ("字节顺序(0:big-endian, network order)")) -> ()  [unwired: 3 in, 3 out]
                                }
                                frame #1 {
                                # "清空操作"
                                n405 = local read "graph_ref"() -> (w437:refnum<vi>[])
                                n406 = local read "path_ref"() -> (w435:refnum<vi>[])
                                n407 = local read "str_ref"() -> (w436:refnum<vi>[])
                                n408 = call "_wmg_newfixture_init.vi"("path_ref"=w435, "graph_ref"=w437, "str_ref"=w436) -> ()  [unwired: 1 in]
                                }
                                }
                                }
                                }
                                }
                                }
                              }
                            }
                          }
                          frame True {
                            n409 = One Button Dialog(message="S4P至少要一个不为空！" ("消息")) -> ()  [unwired: 1 in, 1 out]
                          }
                        }
                      }
                    }
                  }
                }
              }
            }
          }
          event "Import_FixS4P": Value Change {
            n410 = event-data() -> ()  [unwired: 1 in, 5 out]
            n411 = stacked-sequence {
              frame #0 {
              }
            }
          }
          event Panel Close {
            n412 = event-data() -> ()  [unwired: 1 in, 3 out]
          }
        }
      }
    }
  }
